vi "Initialize Hardware References.vi"(8 "error in (no error)":errorcluster, 11 "Hardware Resources in":T1={"VISA resource name"="", "DAQ Type"=0, "Channel 1"={"Acquiring"=FALSE, "Enabled"=FALSE, "Terminal configuration"=32767, "Range"=0, "Coupling"=0}, "Channel 2"={"Acquiring"=FALSE, "Enabled"=FALSE, "Terminal configuration"=0, "Range"=0, "Coupling"=0}, "Timing"={"Sample Time [Time Units]"=0, "Actual Sample Time [s]"=0.0, "Samples per Iteration"=0, "Sample Clock Source"=0, "Time Units"=0, "t0"=timestamp(0 s since 1904-01-01)}, "PS Parameters"={"PS handle"=0, "PS Max_adc"=32767, "PS Enabled Array"=[], "PS Device Info"={"Driver Version"="", "USB Version"="", "Hardware"="", "Variant"="", "Batch and Serial"="", "Cal Date"="", "Kernel Version"="", "Digital HW Version"="", "Analogue HW Version"="", "Firmware 1"="", "Firmware 2"="", "MSO"=FALSE, "Number of Channels"=0}, "Channel 1 Buffer"=refnum, "Channel 2 Buffer"=refnum, "Resolution"=0, "USB Power"=FALSE}, "Trigger"={"Direction"=0, "Threshold [V]"=0.0, "Enabled"=FALSE, "Trigger Source"=0}, "Keithley Parameters"={"Previous End / Current Start"=0, "Quantity"=0}} {"Keithley Parameters"."Quantity" items=["Current", "Voltage"]; "Trigger"."Trigger Source" items=["Channel 1"=0, "Channel 2"=1, "Ext."=4]; "Trigger"."Direction" items=["Falling", "Rising"]; "PS Parameters"."Resolution" items=["8", "12", "14", "15", "16"]; "Timing"."Time Units" items=["Seconds"]; "Timing"."Sample Clock Source" items=["Internal", "External"]; "Channel 2"."Coupling" items=["AC", "DC"]; "Channel 2"."Range" items=["0.01", "0.02", "0.05", "0.1", "0.2", "0.5", "1", "2", "5", "10", "20", "50", "100", "1000"]; "Channel 2"."Terminal configuration" items=["Referenced Single Ended", "Differential"]; "Channel 1"."Coupling" items=["AC", "DC"]; "Channel 1"."Range" items=["0.01", "0.02", "0.05", "0.1", "0.2", "0.5", "1", "2", "5", "10", "20", "50", "100", "1000"]; "Channel 1"."Terminal configuration" items=["Referenced Single Ended", "Differential"]; "DAQ Type" items=["Simulated", "Tektronics DPO2k/3k/4k", "PicoScope 2000a Series", "Keithley DMM7510", "PicoScope 5000a Series", "Arduino"]}) -> (0 "error out":errorcluster, 3 "Hardware Resources out":T1={"VISA resource name"="", "DAQ Type"=0, "Channel 1"={"Acquiring"=FALSE, "Enabled"=FALSE, "Terminal configuration"=32767, "Range"=0, "Coupling"=0}, "Channel 2"={"Acquiring"=FALSE, "Enabled"=FALSE, "Terminal configuration"=0, "Range"=0, "Coupling"=0}, "Timing"={"Sample Time [Time Units]"=0, "Actual Sample Time [s]"=0.0, "Samples per Iteration"=0, "Sample Clock Source"=0, "Time Units"=0, "t0"=timestamp(0 s since 1904-01-01)}, "PS Parameters"={"PS handle"=0, "PS Max_adc"=32767, "PS Enabled Array"=[], "PS Device Info"={"Driver Version"="", "USB Version"="", "Hardware"="", "Variant"="", "Batch and Serial"="", "Cal Date"="", "Kernel Version"="", "Digital HW Version"="", "Analogue HW Version"="", "Firmware 1"="", "Firmware 2"="", "MSO"=FALSE, "Number of Channels"=0}, "Channel 1 Buffer"=refnum, "Channel 2 Buffer"=refnum, "Resolution"=0, "USB Power"=FALSE}, "Trigger"={"Direction"=0, "Threshold [V]"=0.0, "Enabled"=FALSE, "Trigger Source"=0}, "Keithley Parameters"={"Previous End / Current Start"=0, "Quantity"=0}} {"Keithley Parameters"."Quantity" items=["Current", "Voltage"]; "Trigger"."Trigger Source" items=["Channel 1"=0, "Channel 2"=1, "Ext."=4]; "Trigger"."Direction" items=["Falling", "Rising"]; "PS Parameters"."Resolution" items=["8", "12", "14", "15", "16"]; "Timing"."Time Units" items=["Seconds"]; "Timing"."Sample Clock Source" items=["Internal", "External"]; "Channel 2"."Coupling" items=["AC", "DC"]; "Channel 2"."Range" items=["0.01", "0.02", "0.05", "0.1", "0.2", "0.5", "1", "2", "5", "10", "20", "50", "100", "1000"]; "Channel 2"."Terminal configuration" items=["Referenced Single Ended", "Differential"]; "Channel 1"."Coupling" items=["AC", "DC"]; "Channel 1"."Range" items=["0.01", "0.02", "0.05", "0.1", "0.2", "0.5", "1", "2", "5", "10", "20", "50", "100", "1000"]; "Channel 1"."Terminal configuration" items=["Referenced Single Ended", "Differential"]; "DAQ Type" items=["Simulated", "Tektronics DPO2k/3k/4k", "PicoScope 2000a Series", "Keithley DMM7510", "PicoScope 5000a Series", "Arduino"]})   [LabVIEW 2017, in "Acquisition.lvlib"]
doc: "Initialize the hardware references."
uses:
  Acquisition.lvlib
  Hardware Configuration.ctl
  Signal Type.ctl
  Settings/Terminal Configuration.ctl
  Settings/Range.ctl
  Settings/Coupling.ctl
  Settings/Sampling Clock Source.ctl
  Settings/Time Units.ctl
  Settings/Resolution.ctl
  Settings/Trigger Direction.ctl
  Settings/Trigger Source.ctl
  Settings/Quantity.ctl
  <vilib>/Instr/_visa.llb/VISA Configure Serial Port (Instr).vi
  support/DAQ Drivers/Tektronix DPO MSO 2000 4000 Series/Tektronix DPO MSO 2000 4000 Series.lvlib
  support/DAQ Drivers/Keithley DMM7510/Keithley DMM7510.lvlib
  Settings/Settings.lvlib
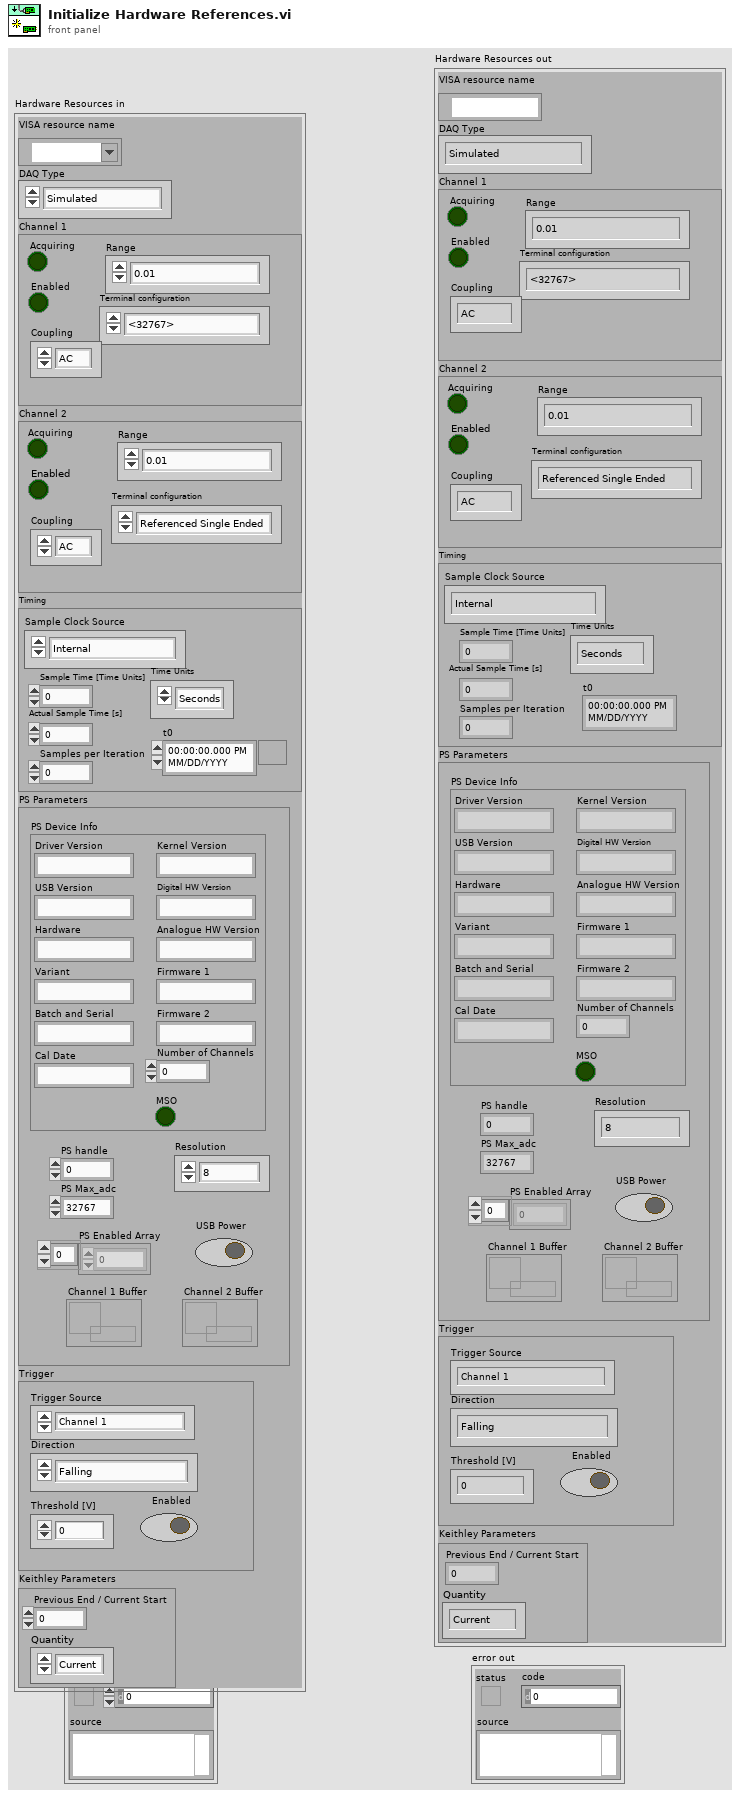
[diagram p1: front panel]
types:
  T1 = typedef "Acquisition.lvlib/Hardware Configuration.ctl" = cluster{"VISA resource name":refnum<visa-resource-name>, "DAQ Type":T2, "Channel 1":cluster{"Acquiring":bool, "Enabled":bool, "Terminal configuration":T3, "Range":T4, "Coupling":T5}, "Channel 2":cluster{"Acquiring":bool, "Enabled":bool, "Terminal configuration":T3, "Range":T4, "Coupling":T5}, "Timing":cluster{"Sample Time [Time Units]":u32, "Actual Sample Time [s]":dbl, "Samples per Iteration":u32, "Sample Clock Source":T6, "Time Units":T7, "t0":timestamp}, "PS Parameters":cluster{"PS handle":i16, "PS Max_adc":i16, "PS Enabled Array":i16[], "PS Device Info":cluster{"Driver Version":string, "USB Version":string, "Hardware":string, "Variant":string, "Batch and Serial":string, "Cal Date":string, "Kernel Version":string, "Digital HW Version":string, "Analogue HW Version":string, "Firmware 1":string, "Firmware 2":string, "MSO":bool, "Number of Channels":i16}, "Channel 1 Buffer":refnum<data-value>, "Channel 2 Buffer":refnum<data-value>, "Resolution":T8, "USB Power":bool}, "Trigger":cluster{"Direction":T9, "Threshold [V]":dbl, "Enabled":bool, "Trigger Source":T10}, "Keithley Parameters":cluster{"Previous End / Current Start":i32, "Quantity":T11}}
  T2 = typedef "Acquisition.lvlib/Signal Type.ctl" = u16
  T3 = typedef "Settings.lvlib/Terminal Configuration.ctl" = u16
  T4 = typedef "Settings.lvlib/Range.ctl" = u16
  T5 = typedef "Settings.lvlib/Coupling.ctl" = i16
  T6 = typedef "Settings.lvlib/Sampling Clock Source.ctl" = u16
  T7 = typedef "Settings.lvlib/Time Units.ctl" = u32
  T8 = typedef "Settings.lvlib/Resolution.ctl" = i32
  T9 = typedef "Settings.lvlib/Trigger Direction.ctl" = u16
  T10 = typedef "Settings.lvlib/Trigger Source.ctl" = u16
  T11 = typedef "Settings.lvlib/Quantity.ctl" = u16
  T12 = cluster{"PS handle":i16, "PS Max_adc":i16, "PS Enabled Array":i16[], "PS Device Info":cluster{"Driver Version":string, "USB Version":string, "Hardware":string, "Variant":string, "Batch and Serial":string, "Cal Date":string, "Kernel Version":string, "Digital HW Version":string, "Analogue HW Version":string, "Firmware 1":string, "Firmware 2":string, "MSO":bool, "Number of Channels":i16}, "Channel 1 Buffer":refnum<data-value>, "Channel 2 Buffer":refnum<data-value>, "Resolution":T8, "USB Power":bool}
  T13 = cluster{"Driver Version":string, "USB Version":string, "Hardware":string, "Variant":string, "Batch and Serial":string, "Cal Date":string, "Kernel Version":string, "Digital HW Version":string, "Analogue HW Version":string, "Firmware 1":string, "Firmware 2":string, "MSO":bool, "Number of Channels":i16}
  T14 = cluster{"Driver Version":string, "USB Version":string, "Hardware":string, "Variant":string, "Batch and Serial":string, "Cal Date":string, "Kernel Version":string, "Digital HW Version":string, "Analogue HW Version":string, "Firmware 1":string, "Firmware 2":string}
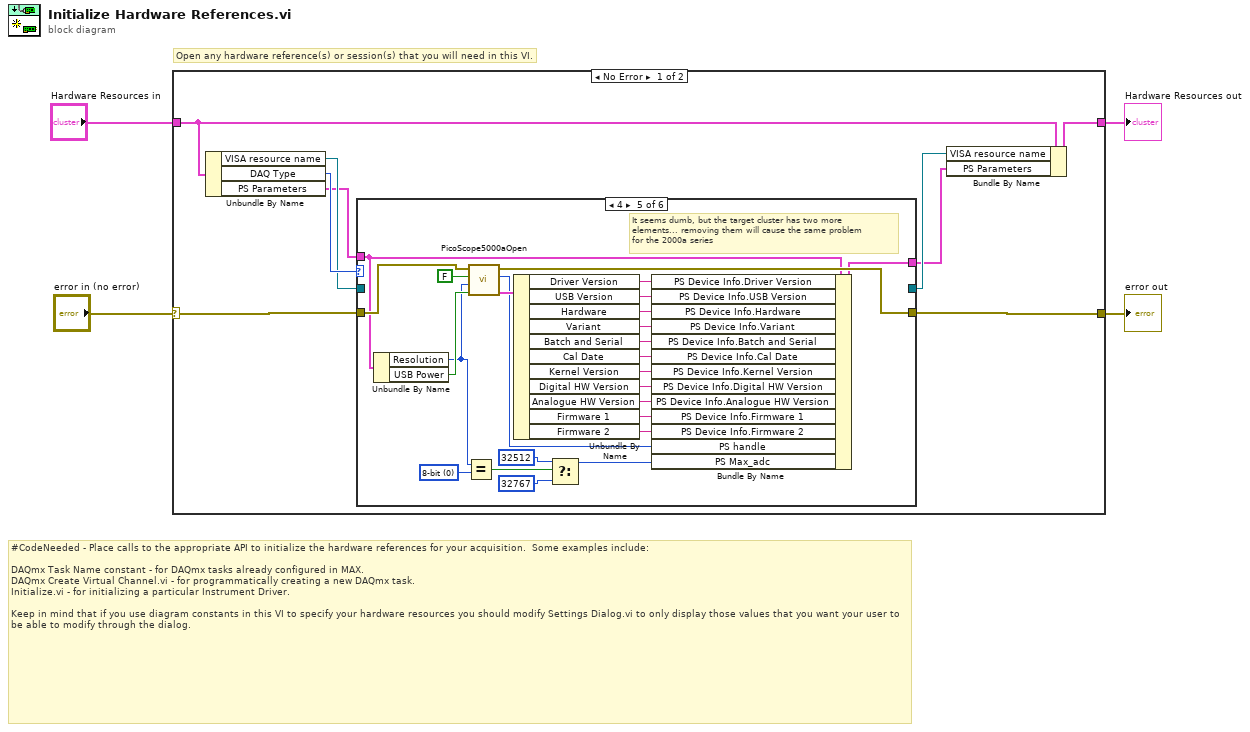
[diagram p0: block diagram]
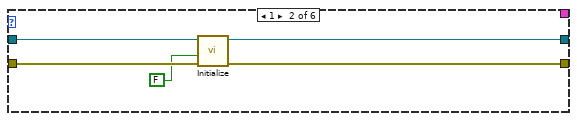
[diagram p3: hidden frame]
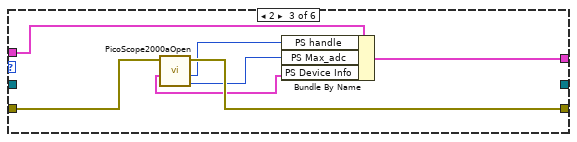
[diagram p4: hidden frame]
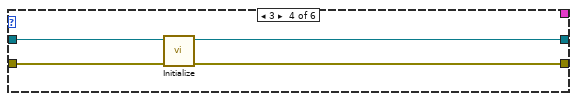
[diagram p5: hidden frame]
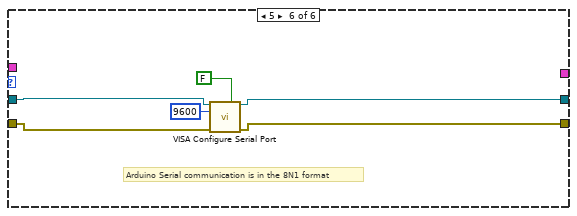
[diagram p6: hidden frame]
diagram:
  # "Open any hardware reference(s) or session(s) that you will need in this VI."
  # "#CodeNeeded - Place calls to the appropriate API to initialize the hardware references for your acquisition.  Some examples include:\n\nDAQmx Task Name constant - for DAQmx tasks already configured in MAX.\nDAQmx Create Virtual Channel.vi - for programmatically creating a new DAQmx task.\nInitialize.vi - for initializing a particular Instrument Driver.\n\nKeep in mind that if you use diagram constants in this VI to specify your hardware resources you should modify Settings Dialog.vi to only display those values that you want your user to be able to modify through the dialog."
  n1 = case shown="No Error" "error in (no error)" {
    selector: "error in (no error)" -> [w10 w63]
    tunnel: [w9 w63] -> w3
    tunnel: "Hardware Resources in" -> [w12 w64]
    tunnel: [w13 w64] -> w1
    frame No Error {
      n2 = Unbundle By Name(w12) -> ("VISA resource name"=w8:refnum<visa-resource-name>, "DAQ Type"=w11:T2, "PS Parameters"=w6:T12)
      n3 = case shown="4" w11 {
        tunnel: w10 -> [w14 w20 w26 w30 w56 w62]
        tunnel: [w14 w19 w27 w28 w55 w57] -> w9
        tunnel: w8 -> [w15 w18 _ w31 _ w60]
        tunnel: [w15 w17 _ w29 _ w58] -> w7
        tunnel: w6 -> [_ _ w25 _ w34 _]
        tunnel: [_ _ w21 _ w41 _] -> w5
        frame 0, Default {
        }
        frame 1 {
          n4 = call "Initialize.vi"("error in (no error)"=w20, "Reset (True)"=FALSE, "VISA resource name"=w18) -> ("error out"=w19:errorcluster, "VISA resource name out"=w17:refnum<visa-resource-name>)  [unwired: 7 in]
        }
        frame 2 {
          n5 = call "PicoScope2000aOpen.vi"("error in (no error)"=w26) -> ("Max Adc value"=w23:i16, "handle"=w24:i16, "error out"=w27:errorcluster, "Device Info"=w22:T13)  [unwired: 3 in]
          n6 = Bundle By Name(cluster=w25, "PS handle"=w24, "PS Max_adc"=w23, "PS Device Info"=w22) -> (w21:T12)
        }
        frame 3 {
          n7 = call "Initialize.vi"("error in (no error)"=w30, "VISA resource name"=w31) -> ("error out"=w28:errorcluster, "VISA resource name out"=w29:refnum<visa-resource-name>)  [unwired: 8 in]
        }
        frame 4 {
          w36 = T8 0 items=["8-bit", "12-bit", "14-bit", "15-bit (max. 2 ch.)", "16-bit (max. 1 ch.)"] ("Resolution")
          # "It seems dumb, but the target cluster has two more\nelements... removing them will cause the same problem\nfor the 2000a series"
          n8 = Unbundle By Name(w34) -> ("Resolution"=w32:T8, "USB Power"=w33:bool)
          n9 = Equal?(x=w32, y=w36) -> (x = y?=w35:bool)
          n10 = call "PicoScope5000aOpen.vi"("USB Powered Selection"=w33, "Resolution"=w32, "Use Serial Number"=FALSE, "error in (no error)"=w56) -> ("Unit Info"=w54:T14, "handle"=w40:i16, "error out"=w55:errorcluster)  [unwired: 2 in, 1 out]
          n11 = Unbundle By Name(w54) -> ("Driver Version"=w53:string, "USB Version"=w52:string, "Hardware"=w51:string, "Variant"=w50:string, "Batch and Serial"=w49:string, "Cal Date"=w48:string, "Kernel Version"=w47:string, "Digital HW Version"=w46:string, "Analogue HW Version"=w45:string, "Firmware 1"=w44:string, "Firmware 2"=w43:string)
          n12 = Select(t=i16 32512, s=w35, f=i16 32767) -> (s? t:f=w39:i16)
          n13 = Bundle By Name(cluster=w34, "PS Device Info.Driver Version"=w53, "PS Device Info.USB Version"=w52, "PS Device Info.Hardware"=w51, "PS Device Info.Variant"=w50, "PS Device Info.Batch and Serial"=w49, "PS Device Info.Cal Date"=w48, "PS Device Info.Kernel Version"=w47, "PS Device Info.Digital HW Version"=w46, "PS Device Info.Analogue HW Version"=w45, "PS Device Info.Firmware 1"=w44, "PS Device Info.Firmware 2"=w43, "PS handle"=w40, "PS Max_adc"=w39) -> (w41:T12)
        }
        frame 5 {
          # "Arduino Serial communication is in the 8N1 format"
          n14 = call-poly "VISA Configure Serial Port"("VISA resource name"=w60, "Enable Termination\nChar (T)"=FALSE ("Enable Termination\nChar (T)"), "baud rate (9600)"=u32 9600, "error in (no error)"=w62) -> ("VISA resource name out"=w58:refnum<visa-resource-name>, "error out"=w57:errorcluster)  [unwired: 10 in]
        }
      }
      n15 = Bundle By Name(cluster=w12, "VISA resource name"=w7, "PS Parameters"=w5) -> (w13:T1)
    }
    frame Error {
    }
  }
  "Hardware Resources out" <- w1
  "error out" <- w3
